vi "2dArrayToNx1Array.vi"(8 "error in (no error)":errorcluster, 10 "2D Array":dbl[][](array[numeric]), 11 "MatOper in":refnum<class "MatOper.lvclass">) -> (0 "error out":errorcluster, 2 "nx1 Array":dbl[][](array[numeric]), 3 "MatOper out":refnum<class "MatOper.lvclass">)   [LabVIEW 2016, in "MatOper.lvclass"]
doc: "Transform mxn array to (m*n)x1 array."
uses:
  MatOper.lvclass
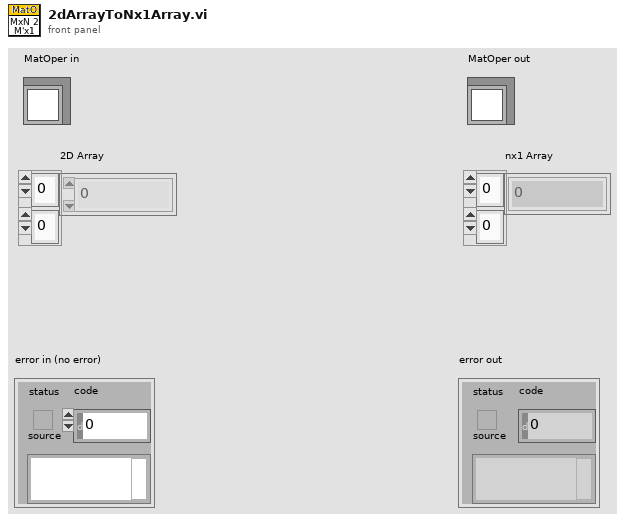
[diagram p1: front panel]
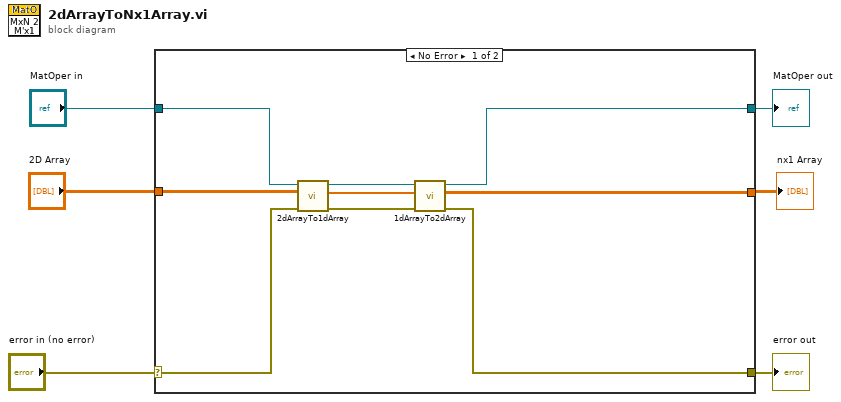
[diagram p0: block diagram]
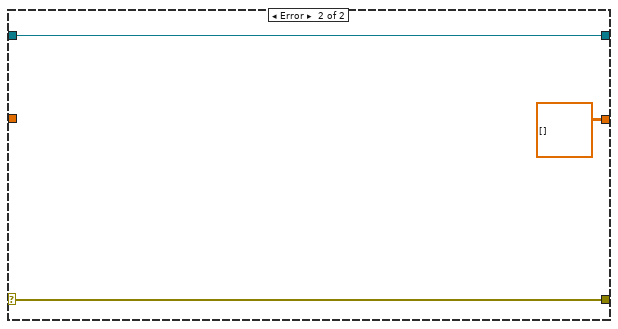
[diagram p2: hidden frame]
diagram:
  n1 = case shown="No Error" "error in (no error)" {
    selector: "error in (no error)" -> [w13 w18]
    tunnel: [w10 w18] -> w5
    tunnel: [w7 w17] -> w3
    tunnel: "MatOper in" -> [w9 w17]
    tunnel: "2D Array" -> [w15 _]
    tunnel: [w14 dbl[][] [] ("2D Array")] -> w1
    frame No Error {
      n2 = call "2dArrayTo1dArray.vi"("error in (no error)"=w13, "2D Array"=w15, "MatOper in"=w9) -> ("error out"=w12:errorcluster, "1D Array"=w11:dbl[], "MatOper out"=w8:refnum<class "MatOper.lvclass">)  [unwired: 6 in]
      n3 = call "1dArrayTo2dArray.vi"("error in (no error)"=w12, "1D Array"=w11, "MatOper in"=w8) -> ("error out"=w10:errorcluster, "2D Array"=w14:dbl[][], "MatOper out"=w7:refnum<class "MatOper.lvclass">)  [unwired: 6 in]
    }
    frame Error {
    }
  }
  "error out" <- w5
  "MatOper out" <- w3
  "nx1 Array" <- w1
